vi "Cfg from FP.vi"(8 "error in (no error)":errorcluster, 11 "Measure Object in":refnum<class "Template Module.lvclass">) -> (0 "error out":errorcluster, 3 "Measure Object out":refnum<class "Template Module.lvclass">)   [LabVIEW 2018, in "Template Module.lvclass"]
uses:
  Template Module.lvclass
  Template Module.lvclass/Template Module.ctl
  Write Configuration.vi
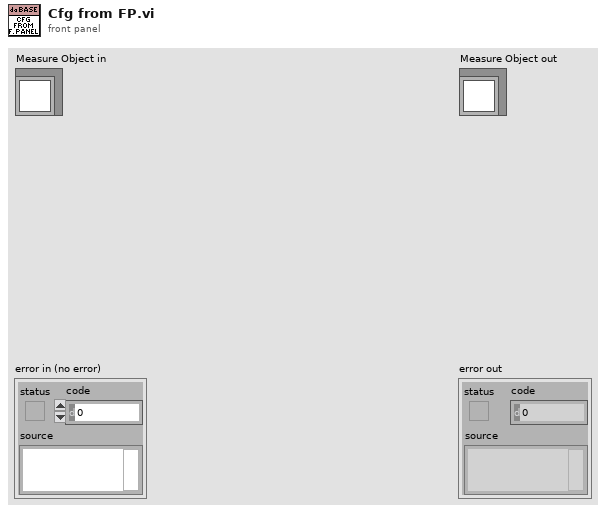
[diagram p1: front panel]
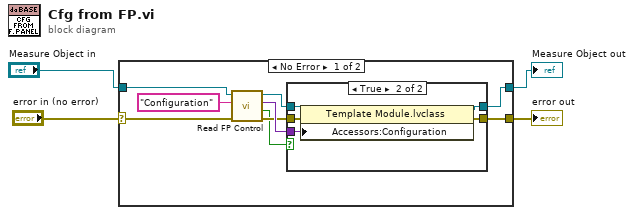
[diagram p0: block diagram]
diagram:
  n1 = case shown="No Error" "error in (no error)" {
    selector: "error in (no error)" -> [w7 w22]
    tunnel: [w6 w22] -> w3
    tunnel: [w10 w21] -> w1
    tunnel: "Measure Object in" -> [w13 w21]
    frame No Error {
      n2 = call-dynamic "Read FP Control.vi"("error in (no error)"=w7, "Control Name"="Configuration", "Measure Object in"=w13) -> ("error out"=w8:errorcluster, "Present"=w5:bool, "Control Value"=w9:variant, "Measure Object out"=w12:refnum<class "Template Module.lvclass">)  [unwired: 5 in]
      n3 = case shown="True" w5 {
        tunnel: w12 -> [w14 w20]
        tunnel: [w14 w19] -> w10
        tunnel: w9 -> [_ w18]
        tunnel: w8 -> [w15 w17]
        tunnel: [w15 w16] -> w6
        frame False {
        }
        frame True {
          n4 = property class="Template Module.lvclass"(reference=w20, error in=w17, "Accessors:Configuration"=w18) -> (reference out=w19:refnum<class "Template Module.lvclass">, error out=w16:errorcluster)
        }
      }
    }
    frame Error {
    }
  }
  "error out" <- w3
  "Measure Object out" <- w1
